vi "File_AddOrUpdatePrefix.vi"(1 "Path":path, 2 "Replace old prefix?":bool, 3 "New Prefix":string, 4 "Old Prefix":string) -> (15 "Path to saved file":path)   [LabVIEW 2010]
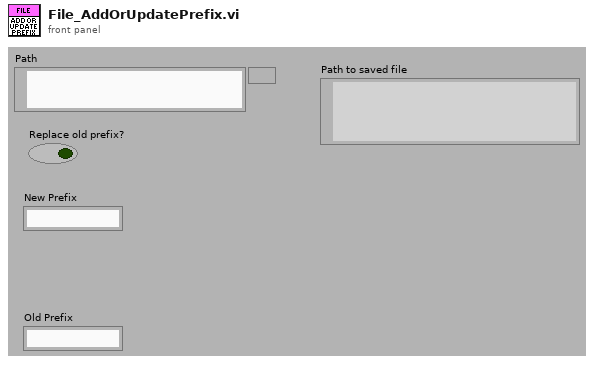
[diagram p1: front panel]
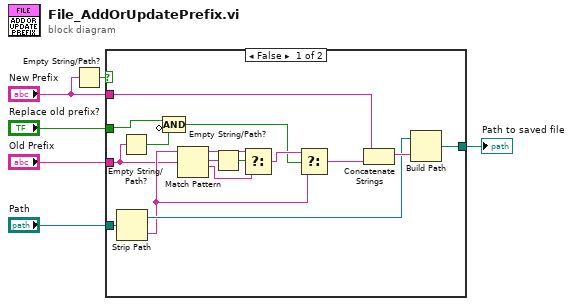
[diagram p0: block diagram]
diagram:
  n1 = Empty String/Path?(string/path="New Prefix") -> (empty?=w2:bool)
  n2 = case shown="False" w2 {
    tunnel: "Replace old prefix?" -> [w8 _]
    tunnel: "Old Prefix" -> [w10 _]
    tunnel: "New Prefix" -> [w16 _]
    tunnel: [w15 w23] -> w4
    tunnel: "Path" -> [w14 w23]
    frame False {
      n3 = Strip Path(path=w14) -> (stripped path=w12:path, name=w11:string)
      n4 = Empty String/Path?(string/path=w10) -> (empty?=w9:bool)
      n5 = Compound Arithmetic op=AND(w8, invert w9) -> (w7:bool)
      n6 = Match Pattern(string=w11, regular expression=w10) -> (before substring=w18:string, match substring=w19:string, after substring=w21:string)  [unwired: 2 out]
      n7 = Empty String/Path?(string/path=w19) -> (empty?=w20:bool)
      n8 = Select(t=w18, s=w20, f=w21) -> (s? t:f=w22:string)
      n9 = Select(t=w22, s=w7, f=w11) -> (s? t:f=w17:string)
      n10 = Concatenate Strings(w16, w17) -> (w13:string)
      n11 = Build Path(base path=w12, name or relative path=w13) -> (appended path=w15:path)
    }
    frame True {
    }
  }
  "Path to saved file" <- w4
